vi "CalculateCounterAndProtections.vi"(8 "error in (no error)":errorcluster, 9 "timeout ms":i32=100, 10 "Async Settings":T1={"Priority"=100, "CAN Session"="", "Frame Count"=0, "Frames"=[]} {"Frames"."Protection Configurations"."CRC Channels"."Data Type" items=["Signed", "Unsigned", "IEEE Float"]}, 11 "Data Refs":T7) -> (0 "error out":errorcluster, 2 "Async Settings":T1={"Priority"=100, "CAN Session"="", "Frame Count"=0, "Frames"=[]} {"Frames"."Protection Configurations"."CRC Channels"."Data Type" items=["Signed", "Unsigned", "IEEE Float"]})   [LabVIEW 2015, in "Protection and Rolling Counter Addon Engine.lvlib"]
uses:
  Protection and Rolling Counter Addon Engine.lvlib
  Types/RT Async Engine Variables.ctl
  Types/RT Frame Settings.ctl
  Types/RT Protection Configuration.ctl
  Shared/Types/Protection Type.ctl
  Shared/Types/InputChannelConfiguration.ctl
  Types/RT Counter Settings.ctl
  Types/RT Data References.ctl
  <vilib>/NI/NIVS Inline Async API/_Data Access Engine/Data Access Engine/Types/Write.DVR.ctl
  <vilib>/NI/NIVS Inline Async API/_Data Access Engine/Access Type Classes/Write/Write.lvclass
  <vilib>/NI/NIVS Inline Async API/_Data Access Engine/Data Access Engine/Types/Read.DVR.ctl
  <vilib>/NI/NIVS Inline Async API/_Data Access Engine/Access Type Classes/Read/Read.lvclass
  <vilib>/NI/NIVS Inline Async API/_Data Access Engine/Access Type Classes/Read/Read.lvclass/Read.ctl
  <vilib>/NI/NIVS Inline Async API/_Data Access Engine/Access Type Classes/Write/Write.lvclass/Write.ctl
  <vilib>/NI/NIVS Inline Async API/_Data Access Engine/Data Access Engine/Methods/Write.Data.Buffer.vi
  <vilib>/NI/NIVS Inline Async API/_Data Access Engine/Data Access Engine/Methods/Write.Data.Commit.vi
  <vilib>/NI/NIVS Inline Async API/_Data Access Engine/Data Access Engine/Methods/Write.Data.vi
  <vilib>/NI/NIVS Inline Async API/_Data Access Engine/Data Access Engine/Methods/Read.Data.vi
  <vilib>/NI/NIVS Inline Async API/_Data Access Engine/Access Type Classes/Write/Write.Buffer.vi
  <vilib>/NI/NIVS Inline Async API/_Data Access Engine/Access Type Classes/Write/Write.Commit.vi
  <vilib>/NI/NIVS Inline Async API/_Data Access Engine/Access Type Classes/Write/Write.ProcessData.vi
  <vilib>/NI/NIVS Inline Async API/_Data Access Engine/Access Type Classes/Read/Read.ProcessData.vi
  <vilib>/xnet/xnet.llb/XNET Write (Frame CAN).vi
  <vilib>/xnet/xnet.llb/XNET Convert (Signal to Frame CAN).vi
  <vilib>/xnet/xnet.llb/XNET Convert (Signal to Frame Raw).vi
  <vilib>/NI/NIVS Inline Async API/_Data Access Engine/Data Access Engine/Data Access Engine.lvclass
  Shared/Protection and Rolling Counter Addon Shared.lvlib
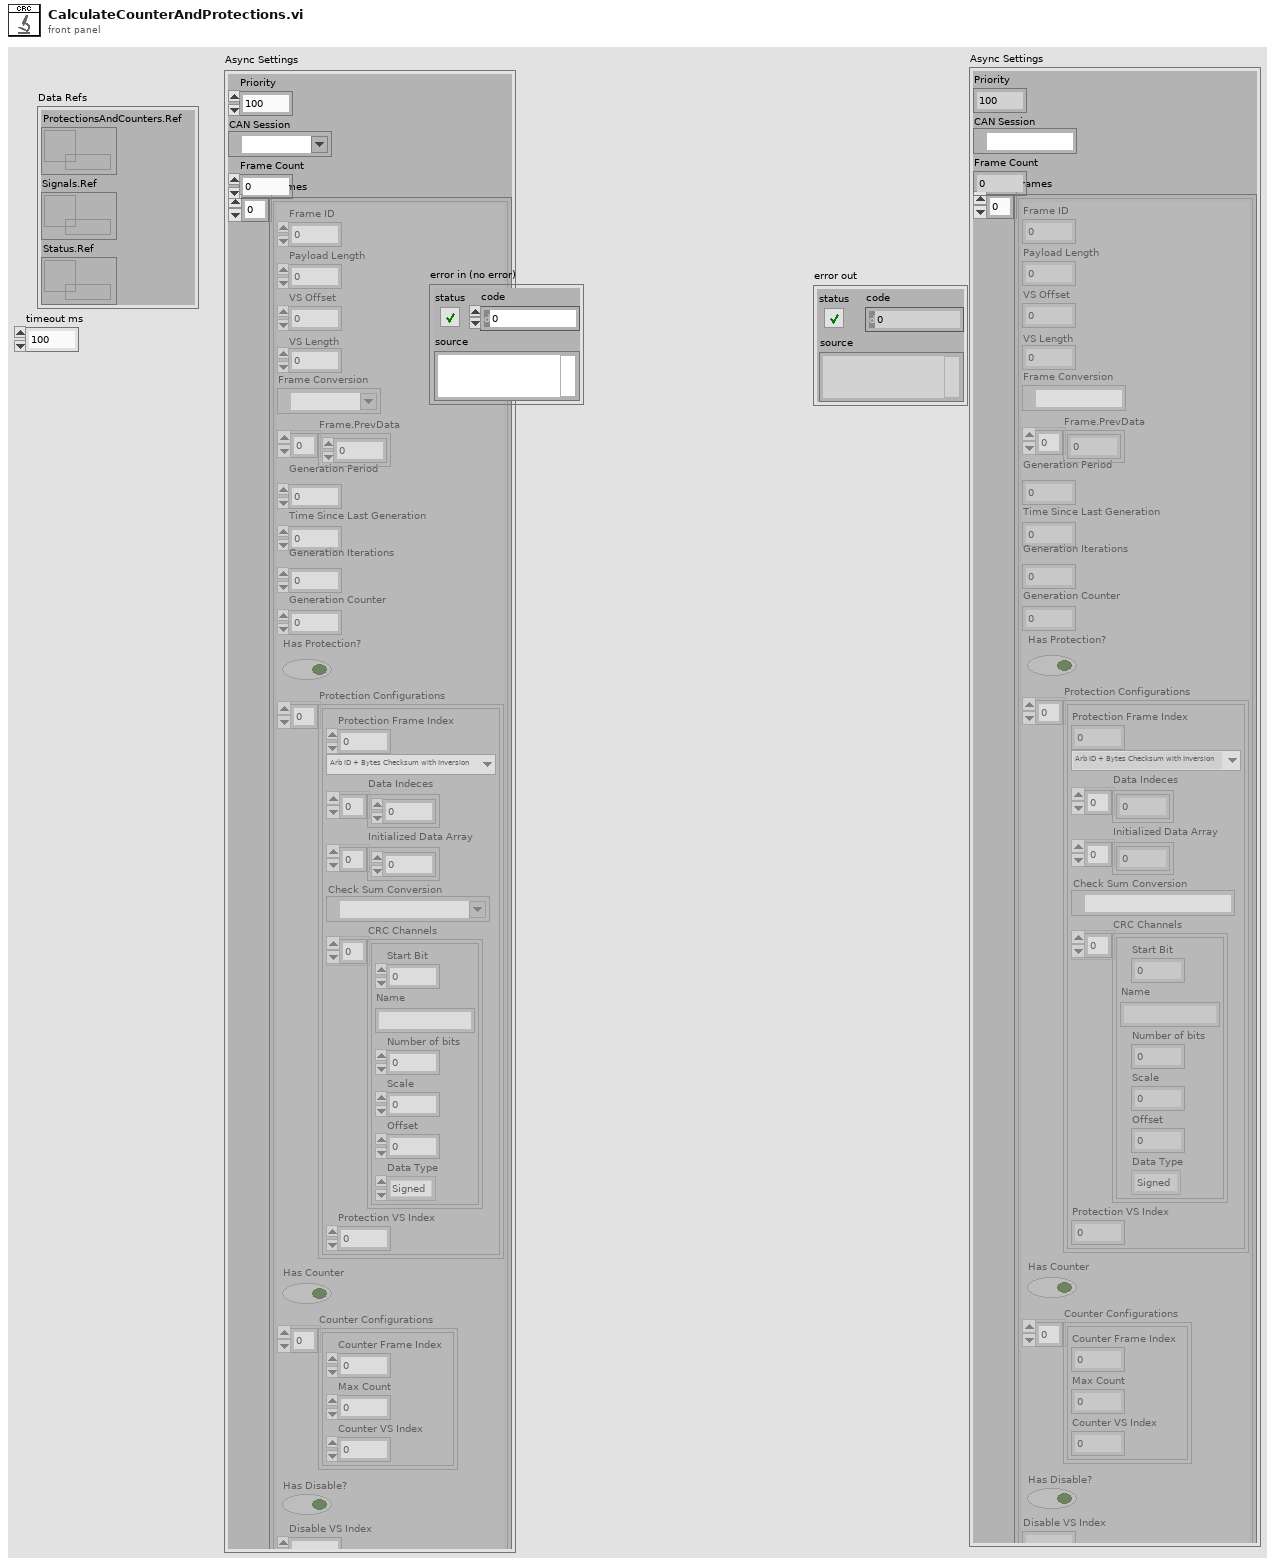
[diagram p1: front panel]
types:
  T1 = typedef "Protection and Rolling Counter Addon Engine.lvlib/RT Async Engine Variables.ctl" = cluster{"Priority":i32, "CAN Session":refnum<k21>, "Frame Count":i32, "Frames":T2[]}
  T2 = typedef "Protection and Rolling Counter Addon Engine.lvlib/RT Frame Settings.ctl" = cluster{"Frame ID":u32, "Payload Length":u32, "VS Offset":i32, "VS Length":i32, "Frame Conversion":refnum<k21>, "Frame.PrevData":dbl[], "Generation Period":u32, "Time Since Last Generation":u32, "Generation Iterations":u32, "Generation Counter":u32, "Has Protection?":bool, "Protection Configurations":T3[], "Has Counter":bool, "Counter Configurations":T6[], "Has Disable?":bool, "Disable VS Index":i32}
  T3 = typedef "Protection and Rolling Counter Addon Engine.lvlib/RT Protection Configuration.ctl" = cluster{"Protection Frame Index":i32, "Protection Type":T4, "Data Indeces":i32[], "Initialized Data Array":dbl[], "Check Sum Conversion":refnum<k21>, "CRC Channels":T5[], "Protection VS Index":i32}
  T4 = typedef "Protection and Rolling Counter Addon Shared.lvlib/Protection Type.ctl" = enum16{"Arb ID + Bytes Checksum with Inversion", "Arb ID + Bytes CRC with Inversion", "Reversed Raw Signal Checksum with Inversion"}
  T5 = typedef "Protection and Rolling Counter Addon Shared.lvlib/InputChannelConfiguration.ctl" = cluster{"Start Bit":i32, "Name":string, "Number of bits":i32, "Scale":dbl, "Offset":dbl, "Data Type":u32}
  T6 = typedef "Protection and Rolling Counter Addon Engine.lvlib/RT Counter Settings.ctl" = cluster{"Counter Frame Index":i32, "Max Count":dbl, "Counter VS Index":i32}
  T7 = typedef "Protection and Rolling Counter Addon Engine.lvlib/RT Data References.ctl" = cluster{"ProtectionsAndCounters.Ref":T8, "Signals.Ref":T9, "Status.Ref":T8}
  T8 = typedef "Data Access Engine.lvlib/Data Access Engine.lvclass/Write.DVR.ctl" = refnum<data-value>
  T9 = typedef "Data Access Engine.lvlib/Data Access Engine.lvclass/Read.DVR.ctl" = refnum<data-value>
  T10 = typedef "XNET Frame CAN.ctl" = cluster{"timestamp":timestamp, "payload":u8[], "identifier":u32, "type":T11, "extended?":bool, "echo?":bool}
  T11 = typedef "XNET Frame Type CAN.ctl" = u8
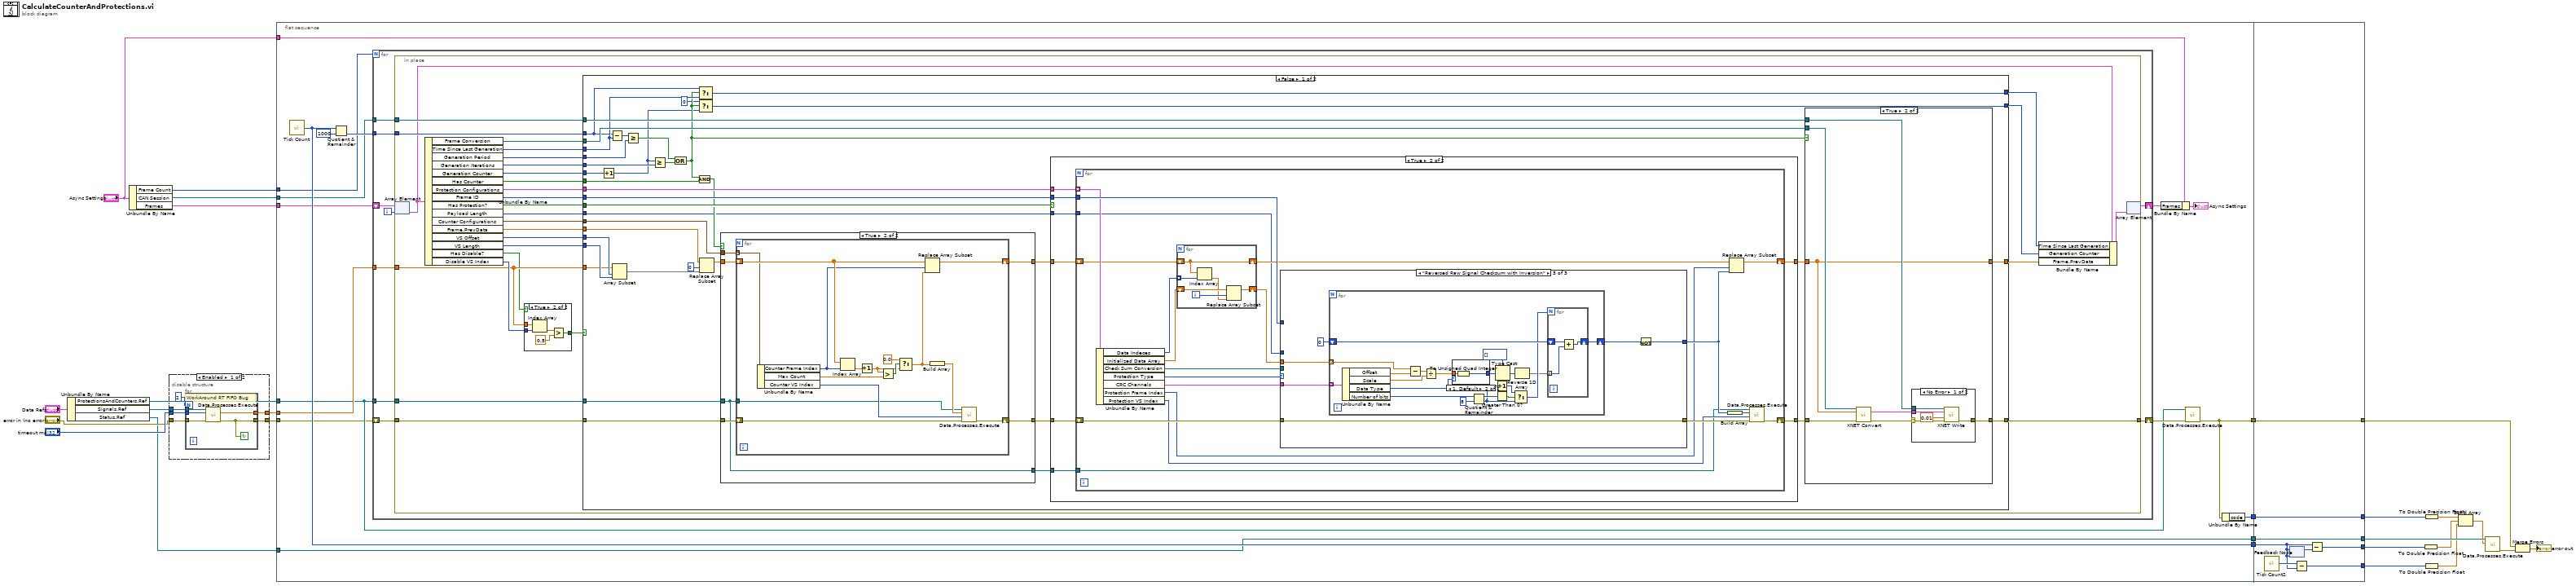
[diagram p0: block diagram]
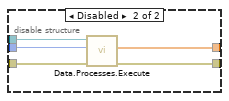
[diagram p2: hidden frame]
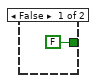
[diagram p3: hidden frame]
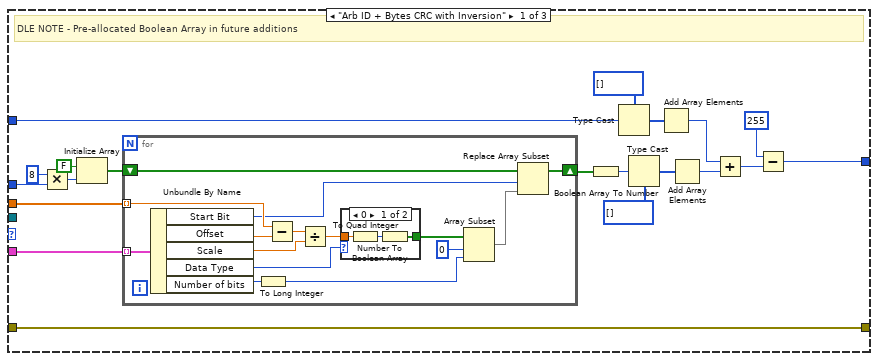
[diagram p6: hidden frame]
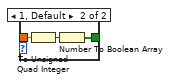
[diagram p7: hidden frame]
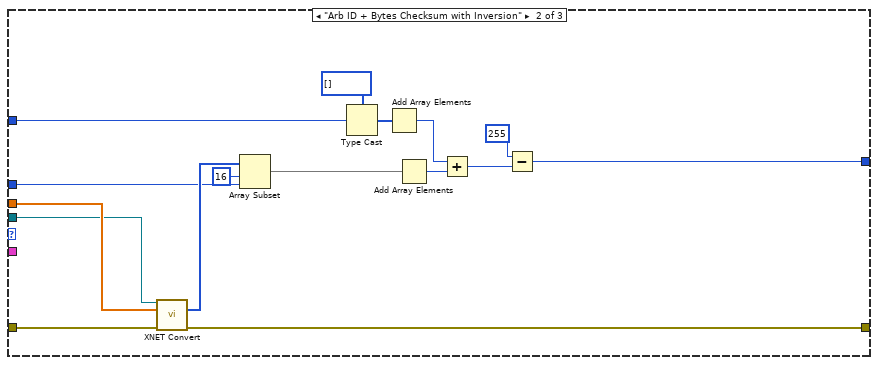
[diagram p8: hidden frame]
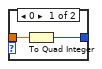
[diagram p9: hidden frame]
diagram:
  n1 = Unbundle By Name("Data Refs") -> ("ProtectionsAndCounters.Ref"=w23:T8, "Signals.Ref"=w15:T9, "Status.Ref"=w16:T8)
  n2 = Unbundle By Name("Async Settings") -> ("Frame Count"=w19:i32, "CAN Session"=w20:refnum<k21>, "Frames"=w21:T2[])
  n3 = disable-structure shown="Enabled" {
    disable-tunnel: "timeout ms" -> [w33 w43]
    disable-tunnel: [w32 w42] -> w24
    disable-tunnel: [w31 w41] -> w22
    disable-tunnel: "error in (no error)" -> [w30 w40]
    disable-tunnel: w15 -> [w29 w39]
    frame Enabled {
      n4 = for {
        N: 2 -> [_]
        tunnel: w33 -> [w38]
        tunnel: [w37] -> w31
        tunnel: w29 -> [w35]
        tunnel: w30 -> [w36]
        tunnel: [w34] -> w32
        stop <- w34 continue-if-true
        # "WorkAround RT FIFO Bug"
        n5 = call-poly <vilib>:"Data.Processes.Execute.vi"("error in (no error)"=w36, "timeout ms"=w38, "Ref"=w35) -> ("error out"=w34:errorcluster, "Values"=w37:dbl[])  [unwired: 6 in, 1 out]
      }
    }
    frame Disabled {
      n6 = call-poly <vilib>:"Data.Processes.Execute.vi"("error in (no error)"=w40, "timeout ms"=w43, "Ref"=w39) -> ("error out"=w42:errorcluster, "Values"=w41:dbl[])  [unwired: 6 in, 1 out]
    }
  }
  n7 = flat-sequence {
    tunnel: [w54] -> w14
    tunnel: [w50] -> w13
    tunnel: [w52] -> w12
    tunnel: [w53] -> w11
    tunnel: w24 -> [w44]
    tunnel: w23 -> [w49]
    tunnel: w22 -> [w51]
    tunnel: w16 -> [w50]
    tunnel: w21 -> [w48]
    tunnel: w20 -> [w47]
    tunnel: w19 -> [w46]
    tunnel: "Async Settings" -> [w45]
    tunnel: [w315] -> w9
    tunnel: [w316] -> w10
    tunnel: [w317] -> w6
    tunnel: w14 -> [w317]
    tunnel: w13 -> [w316]
    tunnel: w12 -> [w310]
    tunnel: [w313] -> w5
    tunnel: [w312] -> w4
    tunnel: w11 -> [w312]
    frame #0 {
      n8 = call "Tick Count"() -> ("Tick Count(uSec)"=w52:u32)
      n9 = Quotient & Remainder(x=w52, y=u32 1000) -> (floor(x/y)=w56:u32)  [unwired: 1 out]
      n10 = for {
        N: w46 -> [_]
        tunnel: w51 -> [w65]
        shift-right: [w67] -> w59
        shift-left: w44 -> [w68]
        tunnel: w56 -> [w66]
        tunnel: w47 -> [w64]
        tunnel: w49 -> [w63]
        shift-right: [w60] -> w58
        shift-left: w48 -> [w62]
        i -> [w61]
        n11 = in-place {
          in-place-border: w68 -> [w96]
          in-place-border: [w95] -> w67
          in-place-border: w66 -> [w91]
          in-place-border: w65 -> [w87]
          in-place-border: w64 -> [w84]
          in-place-border: w63 -> [w81]
          n12 = in-place-array #1(w62, w61) -> (w71:T2)
          n13 = Unbundle By Name(w71) -> ("Frame Conversion"=w89:refnum<k21>, "Time Since Last Generation"=w82:u32, "Generation Period"=w83:u32, "Generation Iterations"=w74:u32, "Generation Counter"=w73:u32, "Has Counter"=w92:bool, "Protection Configurations"=w80:T3[], "Frame ID"=w79:u32, "Has Protection?"=w78:bool, "Payload Length"=w69:u32, "Counter Configurations"=w90:T6[], "Frame.PrevData"=w77:dbl[], "VS Offset"=w94:i32, "VS Length"=w93:i32, "Has Disable?"=w86:bool, "Disable VS Index"=w88:i32)
          n14 = case shown="True" w86 {
            tunnel: w88 -> [_ w102]
            tunnel: w87 -> [_ w101]
            tunnel: [FALSE w99] -> w85
            frame False {
            }
            frame True {
              n15 = Index Array(array=w101, index=w102) -> (element=w100:dbl)
              n16 = Greater?(x=w100, y=0.5 ("x")) -> (0:w99:bool)
            }
          }
          n17 = case shown="False" w85 {
            tunnel: w96 -> [w123 w309]
            tunnel: [w139 w309] -> w95
            tunnel: w94 -> [w138 _]
            tunnel: w93 -> [w137 _]
            tunnel: w92 -> [w136 _]
            tunnel: w91 -> [w113 _]
            tunnel: w83 -> [w125 _]
            tunnel: w90 -> [w135 _]
            tunnel: w80 -> [w133 _]
            tunnel: w78 -> [w132 _]
            tunnel: w79 -> [w131 _]
            tunnel: w89 -> [w129 _]
            tunnel: w87 -> [w128 _]
            tunnel: w84 -> [w127 _]
            tunnel: w82 -> [w114 w308]
            tunnel: w81 -> [w121 _]
            tunnel: w77 -> [w119 w306]
            tunnel: [w115 w306] -> w76
            tunnel: [w112 w308] -> w75
            tunnel: w74 -> [w110 _]
            tunnel: w73 -> [w111 w307]
            tunnel: [w104 w307] -> w72
            tunnel: w69 -> [w103 _]
            frame False {
              n18 = Increment(x=w111) -> (x+1=w106:u32)
              n19 = Subtract(x=w113, y=w114) -> (x-y=w126:u32)
              n20 = Array Subset(array=w128, index=w138, length=w137) -> (w117:dbl[])
              n21 = Greater Or Equal?(x=w126, y=w125) -> (x >= y?=w108:bool)
              n22 = Greater Or Equal?(x=w106, y=w110) -> (x >= y?=w109:bool)
              n23 = Compound Arithmetic op=OR(w108, w109) -> (w107:bool)
              n24 = Select(t=w113, s=w107, f=w114) -> (s? t:f=w112:u32)
              n25 = Select(t=u32 0, s=w107, f=w106) -> (s? t:f=w104:u32)
              n26 = Compound Arithmetic op=AND(w107, w136) -> (w124:bool)
              n27 = Replace Array Subset(array=w119, new element=w117, index=0) -> (w116:dbl[])
              n28 = case shown="True" w124 {
                tunnel: w116 -> [w143 w149]
                tunnel: [w143 w148] -> w134
                tunnel: w135 -> [_ w147]
                tunnel: w123 -> [w142 w146]
                tunnel: [w142 w145] -> w122
                tunnel: w121 -> [w141 w144]
                tunnel: [w141 w144] -> w120
                frame False {
                }
                frame True {
                  n29 = for {
                    shift-right: [w162] -> w148
                    shift-left: w149 -> [w164]
                    tunnel: w147 -> [w161] mode=indexing
                    shift-right: [w151] -> w145
                    shift-left: w146 -> [w152]
                    tunnel: w144 -> [w150]
                    n30 = Unbundle By Name(w161) -> ("Counter Frame Index"=w157:i32, "Max Count"=w163:dbl, "Counter VS Index"=w155:i32)
                    n31 = Index Array(array=w164, index=w157) -> (element=w158:dbl)
                    n32 = Increment(x=w158) -> (x+1=w156:dbl)
                    n33 = Greater?(x=w156, y=w163) -> (0:w160:bool)
                    n34 = Select(t=0.0, s=w160, f=w156) -> (s? t:f=w154:dbl)
                    n35 = Replace Array Subset(array=w164, new element=w154, index=w157) -> (w162:dbl[])
                    n36 = Build Array(w154) -> (w153:dbl[])
                    n37 = call-poly <vilib>:"Data.Processes.Execute.vi"("error in (no error)"=w152, "Offset"=w155, "Values"=w153, "Ref"=w150) -> ("error out"=w151:errorcluster)  [unwired: 7 in]
                  }
                }
              }
              n38 = case shown="True" w132 {
                tunnel: w131 -> [_ w174]
                tunnel: w122 -> [w166 w173]
                tunnel: [w166 w172] -> w140
                tunnel: w134 -> [w165 w171]
                tunnel: w133 -> [_ w170]
                tunnel: [w165 w169] -> w130
                tunnel: w120 -> [_ w168]
                tunnel: w103 -> [_ w167]
                frame False {
                }
                frame True {
                  n39 = for {
                    tunnel: w174 -> [w194]
                    tunnel: w170 -> [w191] mode=indexing
                    shift-right: [w183] -> w172
                    shift-left: w173 -> [w193]
                    shift-right: [w192] -> w169
                    shift-left: w171 -> [w188]
                    tunnel: w168 -> [w176]
                    tunnel: w167 -> [w175]
                    n40 = Unbundle By Name(w191) -> ("Data Indeces"=w189:i32[], "Initialized Data Array"=w186:dbl[], "Check Sum Conversion"=w178:refnum<k21>, "Protection Type"=w179:T4, "CRC Channels"=w190:T5[], "Protection Frame Index"=w177:i32, "Protection VS Index"=w180:i32)
                    n41 = for {
                      shift-right: [w199] -> w187
                      shift-left: w188 -> [w199]
                      tunnel: w189 -> [w200] mode=indexing
                      shift-right: [w195] -> w185
                      shift-left: w186 -> [w198]
                      i -> [w197]
                      n42 = Index Array(array=w199, index=w200) -> (element=w196:dbl)
                      n43 = Replace Array Subset(array=w198, new element=w196, index=w197) -> (w195:dbl[])
                    }
                    n44 = case shown="\"Reversed Raw Signal Checksum with Inversion\"" w179 {
                      tunnel: w194 -> [w218 w255 _]
                      tunnel: [w213 w250 w259] -> w182
                      tunnel: w193 -> [w209 w249 w258]
                      tunnel: [w209 w248 w258] -> w184
                      tunnel: w190 -> [w207 _ w261]
                      tunnel: w185 -> [w208 w245 w260]
                      tunnel: w178 -> [_ w244 _]
                      tunnel: w175 -> [w203 w243 _]
                      frame "Arb ID + Bytes CRC with Inversion" {
                        # "DLE NOTE - Pre-allocated Boolean Array in future additions"
                        n45 = Multiply(x=u32 8, y=w203) -> (x*y=w204:u32)
                        n46 = Initialize Array(FALSE, w204) -> (w206:bool[])
                        n47 = for {
                          tunnel: w207 -> [w235] mode=indexing
                          shift-right: [w226] -> w212
                          shift-left: w206 -> [w228]
                          tunnel: w208 -> [w225] mode=indexing
                          n48 = Unbundle By Name(w235) -> ("Start Bit"=w222:i32, "Offset"=w234:dbl, "Scale"=w232:dbl, "Data Type"=w224:u32, "Number of bits"=w230:i32)
                          n49 = To Long Integer(number=w230) -> (32bit integer=w221:i32)
                          n50 = Subtract(x=w225, y=w234) -> (x-y=w233:dbl)
                          n51 = Divide(x=w233, y=w232) -> (x/y=w231:dbl)
                          n52 = case shown="0" w224 {
                            tunnel: w231 -> [w238 w241]
                            tunnel: [w236 w239] -> w223
                            frame 0 {
                              n53 = To Quad Integer(1:w238) -> (0:w237:i64)
                              n54 = Number To Boolean Array(number=w237) -> (Boolean array=w236:bool[])
                            }
                            frame 1, Default {
                              n55 = To Unsigned Quad Integer(1:w241) -> (0:w240:u64)
                              n56 = Number To Boolean Array(number=w240) -> (Boolean array=w239:bool[])
                            }
                          }
                          n57 = Array Subset(array=w223, index=0, length=w221) -> (w227:bool[])
                          n58 = Replace Array Subset(array=w228, new element=w227, index=w222) -> (w226:bool[])
                        }
                        n59 = Boolean Array To Number(Boolean array=w212) -> (number=w211:u64)
                        n60 = Type Cast(type=u8[] [], x=w218) -> (*(type *) &x=w217:u8[])
                        n61 = Type Cast(type=u8[] [], x=w211) -> (*(type *) &x=w201:u8[])
                        n62 = Add Array Elements(numeric array=w217) -> (sum=w216:u8)
                        n63 = Add Array Elements(numeric array=w201) -> (sum=w220:u8)
                        n64 = Add(x=w216, y=w220) -> (x+y=w215:u8)
                        n65 = Subtract(x=u8 255, y=w215) -> (x-y=w213:u8)
                      }
                      frame "Arb ID + Bytes Checksum with Inversion" {
                        n66 = call-poly <vilib>:"XNET Convert.vi"("session in"=w244, "signal data"=w245, "error in (no error)"=w249) -> ("frame data"=w246:u8[], "error out"=w248:errorcluster)  [unwired: 10 in, 1 out]
                        n67 = Array Subset(array=w246, index=16 ("length"), length=w243) -> (w242:u8[])
                        n68 = Type Cast(type=u8[] [], x=w255) -> (*(type *) &x=w254:u8[])
                        n69 = Add Array Elements(numeric array=w254) -> (sum=w253:u8)
                        n70 = Add Array Elements(numeric array=w242) -> (sum=w257:u8)
                        n71 = Add(x=w253, y=w257) -> (x+y=w252:u8)
                        n72 = Subtract(x=u8 255, y=w252) -> (x-y=w250:u8)
                      }
                      frame "Reversed Raw Signal Checksum with Inversion" {
                        n73 = for {
                          tunnel: w261 -> [w283] mode=indexing
                          tunnel: w260 -> [w280] mode=indexing
                          shift-right: [w277] -> w262
                          shift-left: u8 0 -> [w278]
                          n74 = Unbundle By Name(w283) -> ("Offset"=w282:dbl, "Scale"=w281:dbl, "Data Type"=w279:u32, "Number of bits"=w275:i32)
                          n75 = Subtract(x=w280, y=w282) -> (x-y=w274:dbl)
                          n76 = Divide(x=w274, y=w281) -> (x/y=w273:dbl)
                          n77 = case shown="1, Default" w279 {
                            tunnel: w273 -> [w288 w290]
                            tunnel: [w287 w289] -> w276
                            frame 0 {
                              n78 = To Quad Integer(1:w288) -> (0:w287:i64)
                            }
                            frame 1, Default {
                              n79 = To Unsigned Quad Integer(1:w290) -> (0:w289:u64)
                            }
                          }
                          n80 = Quotient & Remainder(x=w275, y=8) -> (x-y*floor(x/y)=w270:i32, floor(x/y)=w268:i32)
                          n81 = Increment(x=w268) -> (x+1=w269:i32)
                          n82 = Greater Than 0?(x=w270) -> (x > 0?=w271:bool)
                          n83 = Type Cast(type=u8[] [], x=w276) -> (*(type *) &x=w265:u8[])
                          n84 = Select(t=w269, s=w271, f=w268) -> (s? t:f=w267:i32)
                          n85 = Reverse 1D Array(array=w265) -> (reversed array=w264:u8[])
                          n86 = for {
                            N: w267 -> [_]
                            tunnel: w264 -> [w285] mode=indexing
                            shift-right: [w284] -> w277
                            shift-left: w278 -> [w286]
                            n87 = Add(x=w286, y=w285) -> (x+y=w284:u8)
                          }
                        }
                        n88 = Not(x=w262) -> (.not. x?=w259:u8)
                      }
                    }
                    n89 = Build Array(w182) -> (w181:u8[])
                    n90 = Replace Array Subset(array=w187, new element=w182, index=w177) -> (w192:dbl[])
                    n91 = call-poly <vilib>:"Data.Processes.Execute.vi"("error in (no error)"=w184, "Offset"=w180, "Values"=w181, "Ref"=w176) -> ("error out"=w183:errorcluster)  [unwired: 7 in]
                  }
                }
              }
              n92 = case shown="True" w107 {
                tunnel: w140 -> [w292 w298]
                tunnel: [w292 w297] -> w139
                tunnel: w130 -> [w291 w294]
                tunnel: w129 -> [_ w296]
                tunnel: w127 -> [_ w295]
                tunnel: [w291 w294] -> w115
                frame False {
                }
                frame True {
                  n93 = call-poly <vilib>:"XNET Convert.vi"("session in"=w296, "signal data"=w294, "error in (no error)"=w298) -> ("frame data"=w299:T10[], "error out"=w293:errorcluster)  [unwired: 9 in, 2 out]
                  n94 = case shown="No Error" w293 {
                    selector: w293 -> [w301 w305]
                    tunnel: w299 -> [w304 _]
                    tunnel: [w303 w305] -> w297
                    tunnel: w295 -> [w302 _]
                    frame No Error {
                      n95 = call-poly <vilib>:"XNET Write.vi"("session in"=w302, "data"=w304, "timeout (10)"=0.01, "error in (no error)"=w301) -> ("error out"=w303:errorcluster)  [unwired: 10 in, 1 out]
                    }
                    frame Error {
                    }
                  }
                }
              }
            }
            frame True {
            }
          }
          n96 = Bundle By Name(cluster=w71, "Time Since Last Generation"=w75, "Generation Counter"=w72, "Frame.PrevData"=w76) -> (w70:T2)
          n97 = in-place-array #1(w70) -> (w60:T2[])  [unwired: 1 out]
        }
      }
      n98 = Bundle By Name(cluster=w45, "Frames"=w58) -> (→"Async Settings":T1)
      n99 = call-poly <vilib>:"Data.Processes.Execute.vi"("error in (no error)"=w59, "Ref"=w49) -> ("error out"=w54:errorcluster)  [unwired: 9 in]
      n100 = Unbundle By Name(w54) -> ("code"=w53:i32)
    }
    frame #1 {
      n101 = call "Tick Count2"() -> ("Tick Count(uSec)"=w314:u32)
      n102 = feedback #2(w310) -> (w311:u32)
      n103 = feedback-in #2(w310) -> ()
      n104 = Subtract(x=w314, y=w310) -> (x-y=w313:u32)
      n105 = Subtract(x=w310, y=w311) -> (x-y=w315:u32)
    }
  }
  n106 = To Double Precision Float(number=w9) -> (double precision float=w2:dbl)
  n107 = To Double Precision Float(number=w4) -> (double precision float=w3:dbl)
  n108 = To Double Precision Float(number=w5) -> (double precision float=w1:dbl)
  n109 = Build Array(w3, w2, w1) -> (w8:dbl[])
  n110 = call-poly <vilib>:"Data.Processes.Execute.vi"("Values"=w8, "Ref"=w10) -> ("error out"=w7:errorcluster)  [unwired: 9 in]
  n111 = Merge Errors(w6, w7) -> (→"error out":errorcluster)
